vi "Set Footer Object Positions.vi"(4 "FP.width":i16, 5 "SR List.width":u32, 7 "SR List.height":u32, 8 "error in":errorcluster, 10 "label array in":string[](array[string]), 11 "controls[] in":refnum<vi>[](array[refnum])) -> (0 "error out":errorcluster)   [LabVIEW 2018]
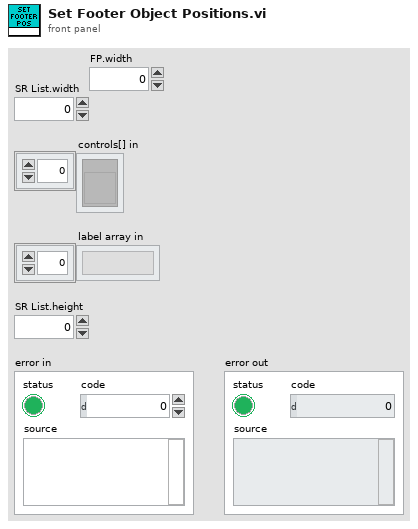
[diagram p1: front panel]
types:
  T1 = typedef "LVRectTypeDef.ctl" = cluster{"Left":i16, "Top":i16, "Right":i16, "Bottom":i16}
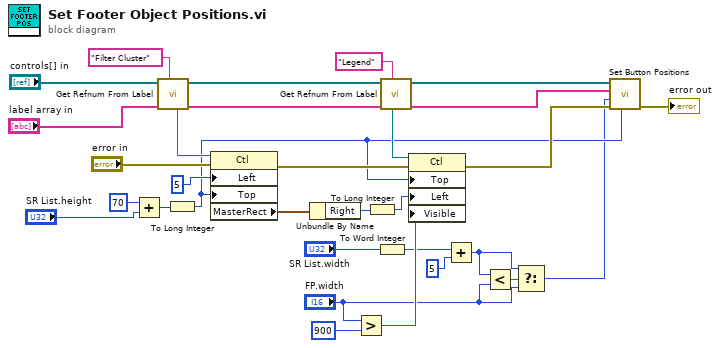
[diagram p0: block diagram]
diagram:
  n1 = Add(x=u32 70, y="SR List.height") -> (x+y=w14:u32)
  n2 = call "Get Refnum From Label.vi"("label"="Filter Cluster" ("element"), "label array in"="label array in", "controls[] in"="controls[] in") -> ("label array out"=w19:string[], "controls[] out"=w17:refnum<vi>[], "refnum out"=w26:refnum<vi>)  [unwired: 6 in]
  n3 = To Long Integer(number=w14) -> (32bit integer=w9:i32)
  n4 = property class="Ctl"(reference=w26, error in="error in", "Left"=5 ("Position:Left"), "Top"=w9) -> (error out=w11:errorcluster, "MasterRect"=w16:T1)  [unwired: 1 out]
  n5 = Unbundle By Name(w16) -> ("Right"=w24:i16)
  n6 = Greater?(x="FP.width", y=u32 900) -> (0:w8:bool)
  n7 = To Long Integer(number=w24) -> (32bit integer=w23:i32)
  n8 = To Word Integer(number="SR List.width") -> (16bit integer=w6:i16)
  n9 = call "Get Refnum From Label.vi"("label"="Legend", "label array in"=w19, "controls[] in"=w17) -> ("label array out"=w20:string[], "controls[] out"=w21:refnum<vi>[], "refnum out"=w18:refnum<vi>)  [unwired: 6 in]
  n10 = property class="Ctl"(reference=w18, error in=w11, "Top"=w9, "Left"=w23, "Visible"=w8) -> (error out=w10:errorcluster)  [unwired: 1 out]
  n11 = Add(x=w6, y=i16 5) -> (x+y=w3:i16)
  n12 = Less?(x=w3, y="FP.width") -> (x < y?=w4:bool)
  n13 = Select(t=w3, s=w4, f="FP.width") -> (s? t:f=w1:i16)
  n14 = call "Set Button Positions.vi"("Top"=w9, "error in"=w10, "Right"=w1, "label array in"=w20, "controls[] in"=w21) -> ("error out"=→"error out":errorcluster)  [unwired: 6 in]
